vi "Find Non-Project Files.vi"() -> ()   [LabVIEW 2020]
uses:
  <vilib>/picture/picture.llb/imagedata.ctl
  Microsoft.VisualBasic
  <resource>/dialog/lvconfig.llb/LV Config Read String.vi
  <vilib>/Utility/lvfile.llb/NI_FileType.lvlib
panel:
  in  "Project":u16(ring)
  in  "Files Not in Project":i32[](listbox) caption="Files Not in Project (these files are on disk under the top-level project folder, but do not exist anywhere within the project)"
  out "FoldersToExclude":string[](array[string])
  in  "Delete Files":bool
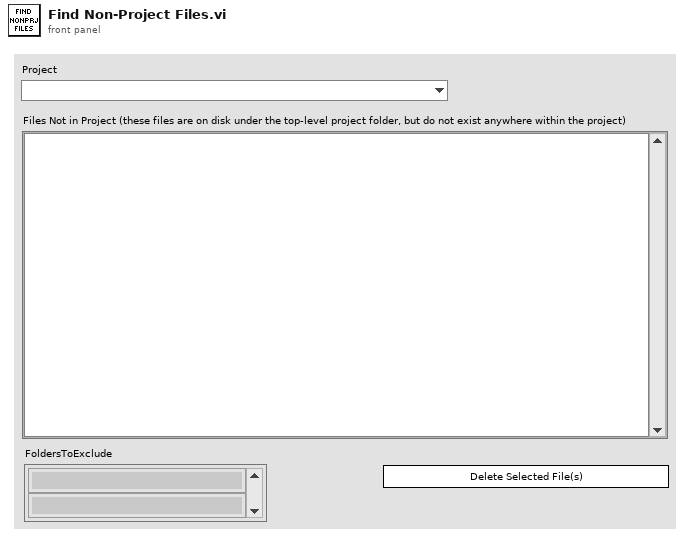
[diagram p1: front panel]
types:
  T1 = enum8{"Enabled", "Disabled", "Disabled and Grayed Out"}
  T2 = typedef "imagedata.ctl" = cluster{"image type":i32, "image depth":i32, "image":u8[], "mask":u8[], "colors":u32[], "Rectangle":cluster{"left":i16, "top":i16, "right":i16, "bottom":i16}}
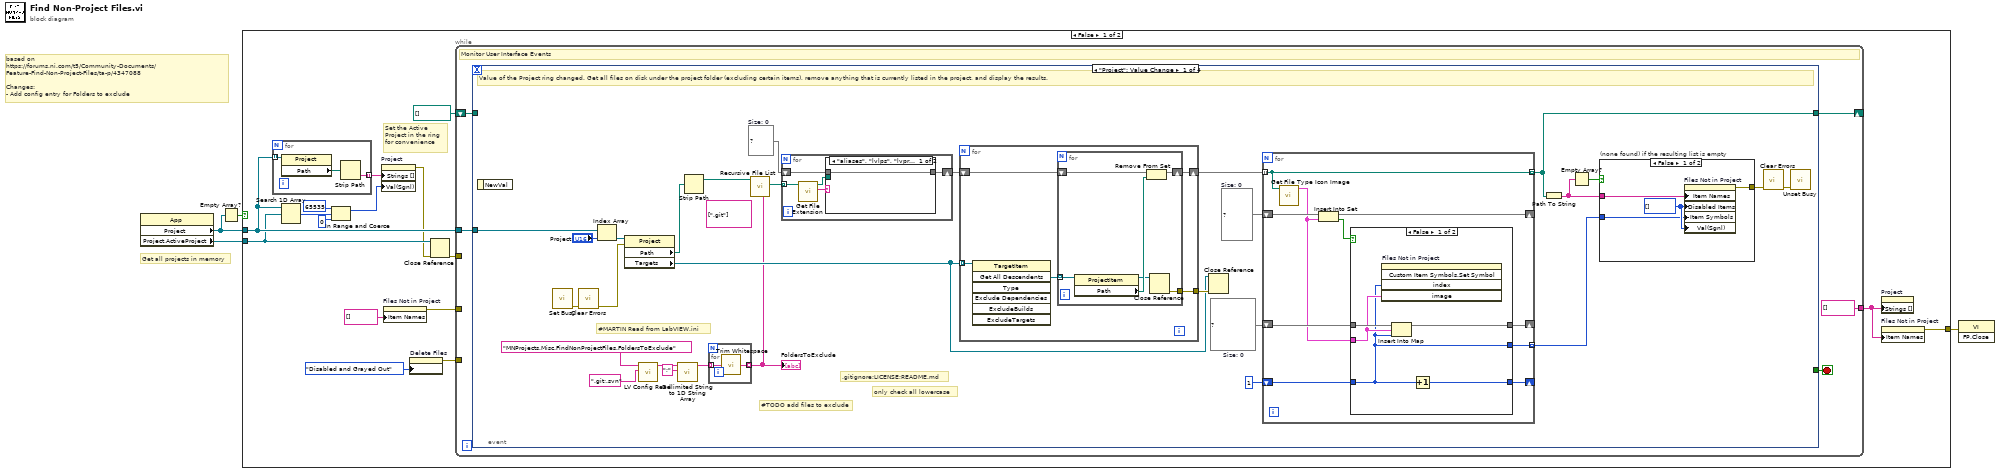
[diagram p0: block diagram]
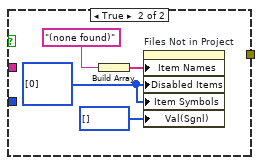
[diagram p2: hidden frame]
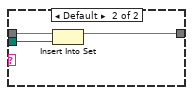
[diagram p3: hidden frame]
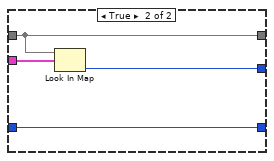
[diagram p4: hidden frame]
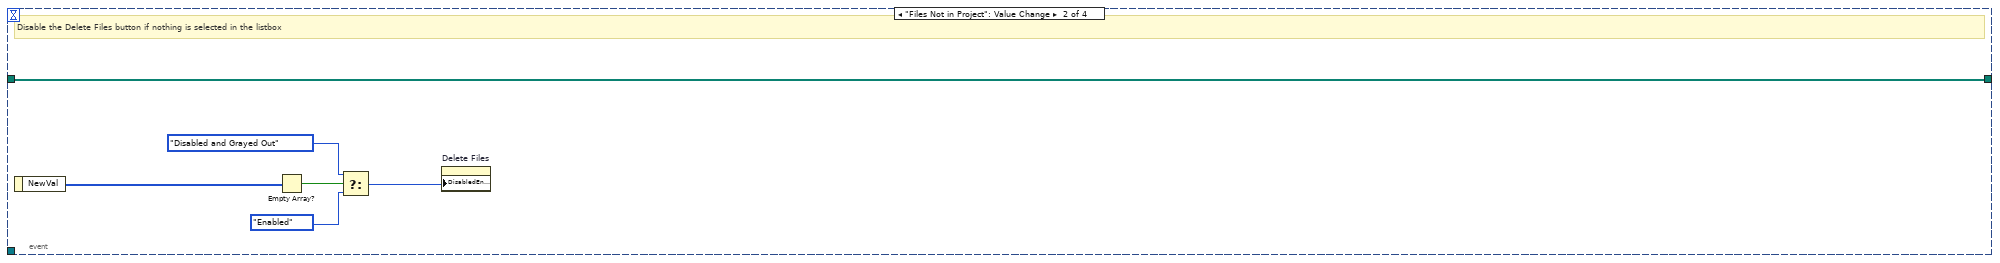
[diagram p5: hidden frame]
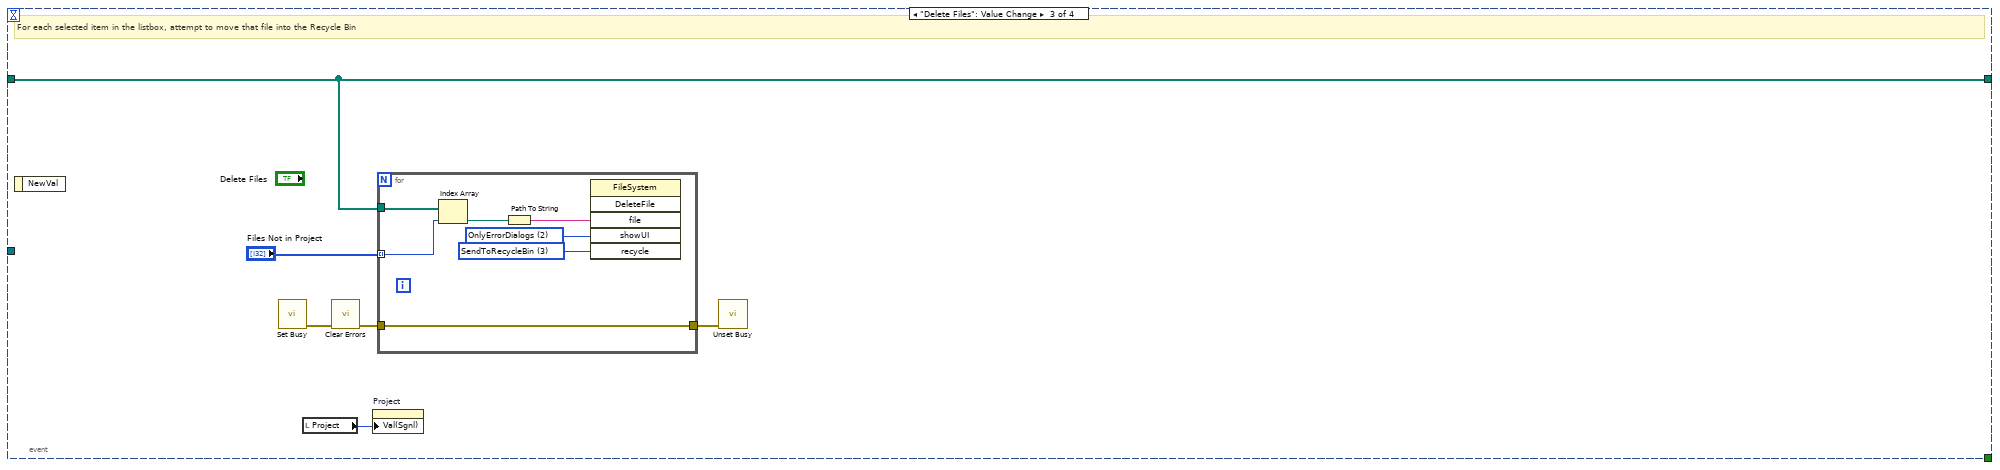
[diagram p6: hidden frame]
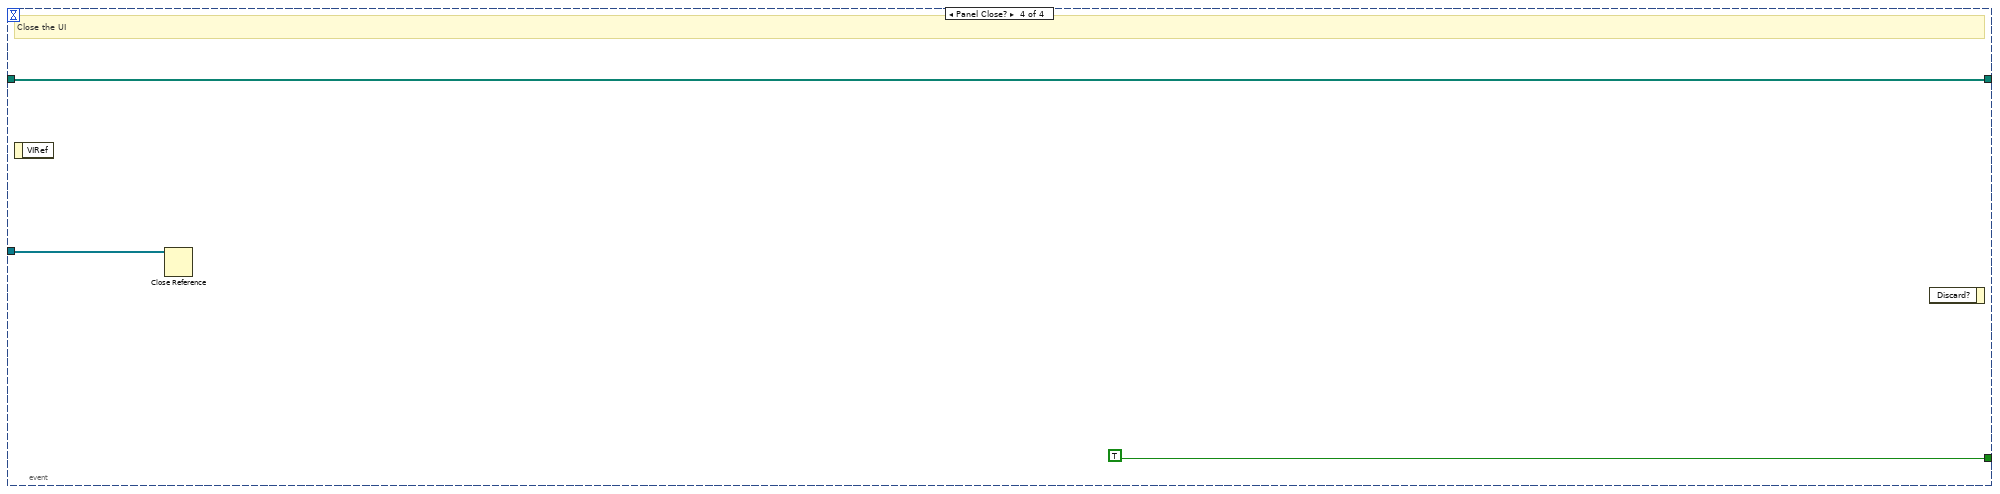
[diagram p7: hidden frame]
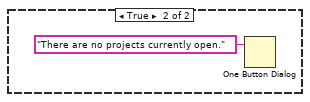
[diagram p8: hidden frame]
diagram:
  # "based on\nhttps://forums.ni.com/t5/Community-Documents/Feature-Find-Non-Project-Files/ta-p/4347088\n\nChanges:\n- Add config entry for Folders to exclude"
  # "Get all projects in memory"
  n1 = property class="App"() -> ("Project"=w3:refnum<vi>[], "Project.ActiveProject"=w4:refnum<vi>)  [unwired: 2 in, 2 out]
  n2 = Empty Array?(array=w3) -> (empty?=w2:bool)
  n3 = case shown="False" w2 {
    tunnel: w3 -> [w18 _]
    tunnel: w4 -> [w17 _]
    tunnel: [w9 _] -> w1
    frame False {
      # "Set the Active Project in the ring for convenience"
      n4 = for {
        tunnel: w18 -> [w23] mode=indexing
        tunnel: [w21] -> w19 mode=indexing
        n5 = property class="Project"(reference=w23) -> ("Path"=w22:path)  [unwired: 1 in, 2 out]
        n6 = Strip Path(path=w22) -> (name=w21:string)  [unwired: 1 out]
      }
      n7 = Search 1D Array(1D array=w18, element=w17) -> (index of element=w8:i32)  [unwired: 1 in]
      n8 = In Range and Coerce(upper limit=65535, x=w8, lower limit=0) -> (coerced(x)=w6:i32)  [unwired: 1 out]
      n9 = property on="Project" class="Ring (strict)"("Strings []"=w19, "Val(Sgnl)"=w6) -> (error out=w16:errorcluster)  [unwired: 2 in, 1 out]
      n10 = property on="Files Not in Project" class="LstBox (strict)"("Item Names"=string[] []) -> (error out=w12:errorcluster)  [unwired: 2 in, 1 out]
      n11 = property on="Delete Files" class="Bool"("DisabledEnum"=T1."Disabled and Grayed Out" ("Disabled")) -> (error out=w13:errorcluster)  [unwired: 2 in, 1 out]
      n12 = Close Reference(reference=w17, error in (no error)=w16) -> (error out=w15:errorcluster)
      n13 = while {
        shift-right: [w28] -> _
        shift-left: path[] [] -> [w27]
        tunnel: w18 -> [w26]
        tunnel: w15 -> [_]
        tunnel: w13 -> [_]
        tunnel: w12 -> [_]
        tunnel: [string[] [] ("Strings []")] -> w10
        stop <- w25 stop-if-true
        # "Monitor User Interface Events"
        n14 = event shown="[0] \"Project\": Value Change" {
          selector: _ -> [_ _ _ _]
          dyn-events: _ -> [_ _ _ _]
          timeout: _ -> [_ _ _ _]
          tunnel: [w51 w111 w117 w127] -> w28
          tunnel: w27 -> [_ w111 w117 w127]
          tunnel: w26 -> [w50 _ _ w125]
          tunnel: [_ _ _ TRUE ("Discard?")] -> w25
          event "Project": Value Change {
            w37 = set{T2} {}  # Size: 0
            w36 = map{T2, i32} {}  # Size: 0
            (unwired) string[] [".git"] ("Folders to Exclude")
            w56 = set{path} {}  # Size: 0
            # "only check all lowercase"
            # ".gitignore;LICENSE;README.md"
            # "#TODO add files to exclude"
            # "#MARTIN Read from LabVIEW.ini"
            # "Value of the Project ring changed. Get all files on disk under the project folder (excluding certain items), remove anything that is currently listed in the project, and display the results."
            n15 = event-data() -> ()  [unwired: 1 in, 1 out]
            n16 = call <vilib>:"Set Busy.vi"() -> ("error out"=w44:errorcluster)  [unwired: 10 in, 1 out]
            n17 = call <vilib>:"Clear Errors.vi"("error in (no error)"=w44) -> ("error out"=w43:errorcluster)  [unwired: 5 in, 1 out]
            n18 = Index Array(array=w50, index="Project") -> (element=w49:refnum<vi>)
            n19 = property class="Project"(reference=w49, error in=w43) -> ("Path"=w52:path, "Targets"=w45:refnum<vi>[])  [unwired: 2 out]
            n20 = call-poly <resource>:"LV Config Read.vi"("default value"=".git;.svn", "key"="MNProjects.Misc.FindNonProjectFiles.FoldersToExclude") -> ("value"=w33:string)  [unwired: 3 in, 2 out]
            n21 = call <vilib>:"Delimited String to 1D String Array.vi"("delimiter"=";", "delimited string"=w33) -> ("string array"=w30:string[])  [unwired: 9 in]
            n22 = Strip Path(path=w52) -> (stripped path=w47:path)  [unwired: 1 out]
            n23 = for {
              tunnel: w30 -> [w58] mode=indexing
              tunnel: [w57] -> w29 mode=indexing
              n24 = call <vilib>:"Trim Whitespace.vi"("string"=w58) -> ("trimmed string"=w57:string)  [unwired: 1 in]
            }
            "FoldersToExclude" <- w29
            n25 = call <vilib>:"Recursive File List.vi"("Folders to Exclude"=w29, "Folder Path"=w47) -> ("All Files in Dir"=w54:path[])  [unwired: 5 in, 4 out]
            n26 = for {
              tunnel: w54 -> [w71] mode=indexing
              shift-right: [w70] -> w55
              shift-left: w56 -> [w69]
              n27 = call <vilib>:"Get File Extension.vi"("file"=w71) -> ("lowercase file extension"=w67:string, "dup file"=w68:path)  [unwired: 6 in, 3 out]
              n28 = case shown="\"aliases\", \"lvlps\", \"lvproj\"" w67 {
                tunnel: [w72 w75] -> w70
                tunnel: w69 -> [w72 w74]
                tunnel: w68 -> [_ w73]
                frame "aliases", "lvlps", "lvproj" {
                }
                frame Default {
                  n29 = Insert Into Set(10:w73, 11:w74) -> (3:w75:set{path})  [unwired: 1 out]
                }
              }
            }
            n30 = for {
              tunnel: w45 -> [w80] mode=indexing
              shift-right: [w77] -> w53
              shift-left: w55 -> [w79]
              tunnel: [w76] -> w46
              n31 = invoke class="TargetItem" method="Get All Descendents"(reference=w80) -> ("All Descendents"=w78:refnum<vi>[])  [unwired: 6 in, 6 out]
              n32 = for {
                tunnel: w78 -> [w86] mode=indexing
                shift-right: [w83] -> w77
                shift-left: w79 -> [w85]
                tunnel: [w81] -> w76
                n33 = property class="ProjectItem"(reference=w86) -> (reference out=w82:refnum<vi>, "Path"=w84:path)  [unwired: 1 in, 1 out]
                n34 = Remove From Set(10:w84, 11:w85) -> (3:w83:set{path})  [unwired: 1 out]
                n35 = Close Reference(reference=w82) -> (error out=w81:errorcluster)  [unwired: 1 in]
              }
            }
            n36 = Close Reference(reference=w45, error in (no error)=w46) -> ()  [unwired: 1 out]
            n37 = for {
              tunnel: w53 -> [w96] mode=indexing
              tunnel: [w96] -> w51 mode=indexing
              shift-right: [w91] -> _
              shift-left: w37 -> [w92]
              shift-right: [w95] -> _
              shift-left: 1 -> [w94]
              shift-right: [w89] -> _
              shift-left: w36 -> [w93]
              tunnel: [w87] -> w35 mode=indexing
              n38 = call <vilib>:"Get File Type Icon Image.vi"("path"=w96) -> ("image data"=w88:T2)  [unwired: 9 in, 1 out]
              n39 = Insert Into Set(10:w88, 11:w92) -> (2:w90:bool, 3:w91:set{T2})
              n40 = case shown="False" w90 {
                tunnel: [w99 w105] -> w95
                tunnel: w94 -> [w97 w105]
                tunnel: w93 -> [w101 w104]
                tunnel: [w100 w104] -> w89
                tunnel: w88 -> [w98 w103]
                tunnel: [w97 w102] -> w87
                frame False {
                  n41 = invoke on="Files Not in Project" class="LstBox (strict)" method="Custom Item Symbols.Set Symbol"("index"=w97, "image"=w98) -> ()  [unwired: 3 in, 5 out]
                  n42 = Insert Into Map(map in=w101, key=w98, value=w97) -> (map out=w100:map{T2, i32})  [unwired: 2 out]
                  n43 = Increment(x=w97) -> (x+1=w99:i32)
                }
                frame True {
                  n44 = Look In Map(map=w104, key=w103) -> (value=w102:i32)  [unwired: 1 in, 1 out]
                }
              }
            }
            n45 = Path To String(path=w51) -> (string=w41:string[])
            n46 = Empty Array?(array=w41) -> (empty?=w40:bool)
            n47 = case "(none found) if the resulting list is empty" shown="False" w40 {
              tunnel: w41 -> [w62 _]
              tunnel: [w60 _] -> w39
              tunnel: w35 -> [w59 _]
              frame False {
                w61 = i32[] [] ("Files")
                n48 = property on="Files Not in Project" class="LstBox (strict)"("Item Names"=w62, "Disabled Items"=w61, "Item Symbols"=w59, "Val(Sgnl)"=w61) -> (error out=w60:errorcluster)  [unwired: 2 in, 1 out]
              }
              frame True {
                w63 = i32[] [0] ("Files")
                n49 = Build Array("(none found)") -> (w66:string[])
                n50 = property on="Files Not in Project" class="LstBox (strict)"("Item Names"=w66, "Disabled Items"=w63, "Item Symbols"=w63, "Val(Sgnl)"=i32[] [] ("Files")) -> ()  [unwired: 2 in, 2 out]
              }
            }
            n51 = call <vilib>:"Clear Errors.vi"("error in (no error)"=w39) -> ("error out"=w42:errorcluster)  [unwired: 5 in, 1 out]
            n52 = call <vilib>:"Unset Busy.vi"("error in (no error)"=w42) -> ()  [unwired: 10 in, 1 out]
          }
          event "Files Not in Project": Value Change {
            # "Disable the Delete Files button if nothing is selected in the listbox"
            n53 = event-data() -> ("NewVal"=w110:i32[])  [unwired: 1 in]
            n54 = Empty Array?(array=w110) -> (empty?=w109:bool)
            n55 = Select(t=T1."Disabled and Grayed Out" ("Disabled"), s=w109, f=T1."Enabled" ("Disabled")) -> (s? t:f=w108:T1)
            n56 = property on="Delete Files" class="Bool"("DisabledEnum"=w108) -> ()  [unwired: 2 in, 2 out]
          }
          event "Delete Files": Value Change {
            # "For each selected item in the listbox, attempt to move that file into the Recycle Bin"
            n57 = event-data() -> ()  [unwired: 1 in, 1 out]
            n58 = call <vilib>:"Set Busy.vi"() -> ("error out"=w114:errorcluster)  [unwired: 10 in, 1 out]
            n59 = local read "Project"() -> (w116:u16)
            n60 = call <vilib>:"Clear Errors.vi"("error in (no error)"=w114) -> ("error out"=w113:errorcluster)  [unwired: 5 in, 1 out]
            n61 = property on="Project" class="Ring (strict)"("Val(Sgnl)"=w116) -> ()  [unwired: 2 in, 2 out]
            n62 = for {
              tunnel: "Files Not in Project" -> [w123] mode=indexing
              tunnel: w117 -> [w124]
              tunnel: [w118] -> w112
              tunnel: w113 -> [w118]
              w119 = 3 items=["DeletePermanently"=2, "SendToRecycleBin"=3] ("recycle")
              w120 = 2 items=["OnlyErrorDialogs"=2, "AllDialogs"=3] ("showUI")
              n63 = Index Array(array=w124, index=w123) -> (element=w122:path)
              n64 = Path To String(path=w122) -> (string=w121:string)
              n65 = invoke class="FileSystem" method="DeleteFile"("file"=w121, "showUI"=w120, "recycle"=w119) -> ()  [unwired: 3 in, 6 out]
            }
            n66 = call <vilib>:"Unset Busy.vi"("error in (no error)"=w112) -> ()  [unwired: 10 in, 1 out]
          }
          event Panel Close? {
            # "Close the UI"
            n67 = event-data() -> ()  [unwired: 1 in, 1 out]
            n68 = Close Reference(reference=w125) -> ()  [unwired: 1 in, 1 out]
            n69 = event-data() -> ()  [unwired: 2 in, 1 out]
          }
        }
      }
      n70 = property on="Project" class="Ring (strict)"("Strings []"=w10) -> ()  [unwired: 2 in, 2 out]
      n71 = property on="Files Not in Project" class="LstBox (strict)"("Item Names"=w10) -> (error out=w9:errorcluster)  [unwired: 2 in, 1 out]
    }
    frame True {
      n72 = One Button Dialog(message="There are no projects currently open.") -> ()  [unwired: 1 in, 1 out]
    }
  }
  n73 = invoke class="VI" method="FP.Close"(error in=w1) -> ()  [unwired: 2 in, 3 out]
